vi "Test Executable.vi"() -> ()   [LabVIEW 2014]
uses:
  Core/LabVIEW CI Service/Classes/LabVIEW Instance/LabVIEW Instance.lvclass
  Dummy Job/Dummy Job.lvclass
  Core/LabVIEW CI Service/Actors/Jobber Proxy/Jobber Proxy/Jobber Proxy.lvclass
  <vilib>/ActorFramework/Actor/Actor.lvclass
  <vilib>/ActorFramework/Message Queue/Message Queue.lvclass
  <vilib>/ActorFramework/Message Dequeuer/Message Dequeuer.lvclass
  <vilib>/ActorFramework/LastAck/Last Ack.lvclass
  Core/LabVIEW CI Service/Classes/Job/Job.lvclass
  Core/LabVIEW CI Service/Controls/Job Results - STYP.ctl
panel:
  out "Boolean":bool
  in  "Wait (ms)":u32=30000
  out "Results":T1 {"Status" items=["Service Error"=504, "Abort"=503, "Fail"=500, "Pass"=200]}
  in  "Launch":bool
  in  "Show Panel":bool=TRUE
  in  "Open":bool
  in  "Port":i32=3366
  in  "Machine Name":string="10.0.19.177"
  in  "stop":bool
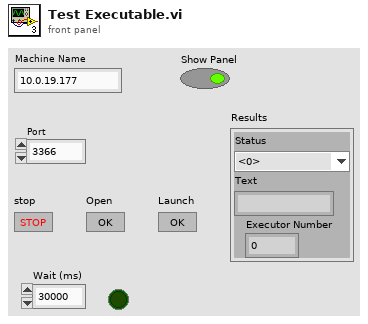
[diagram p1: front panel]
types:
  T1 = typedef "Job Results - STYP.ctl" = cluster{"Status":u16, "Text":string, "Executor Number":i32}
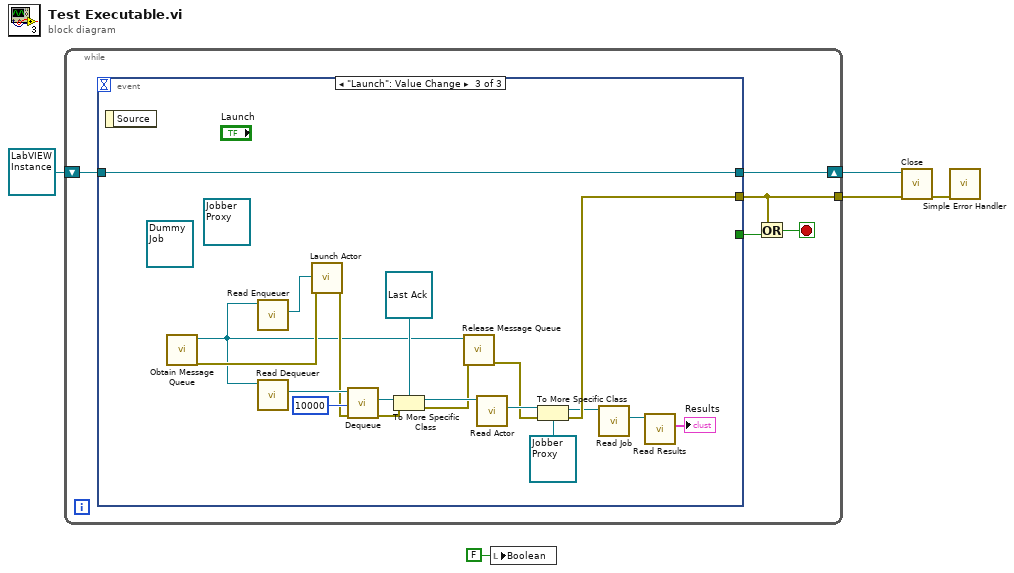
[diagram p0: block diagram]
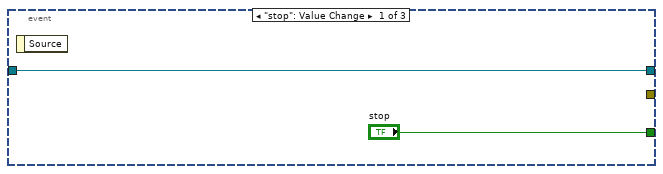
[diagram p2: hidden frame]
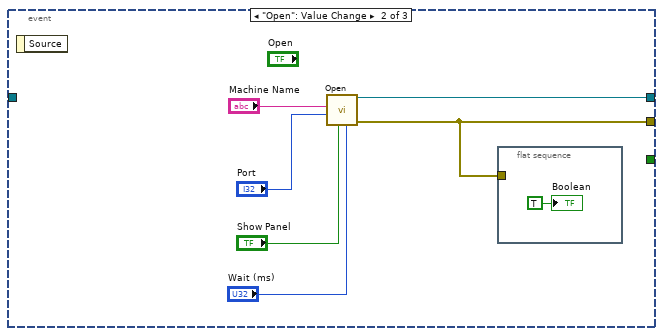
[diagram p3: hidden frame]
diagram:
  n1 = while {
    shift-right: [w9] -> w4
    shift-left: refnum<class "LabVIEW Instance.lvclass"> refnum ("LabVIEW Instance") -> [w10]
    tunnel: [w8] -> w2
    stop <- w7 stop-if-true
    n2 = event shown="[2] \"Launch\": Value Change" {
      selector: _ -> [_ _ _]
      dyn-events: _ -> [_ _ _]
      timeout: _ -> [_ _ _]
      tunnel: w10 -> [w12 _ w38]
      tunnel: [w12 w16 w38] -> w9
      tunnel: [_ w13 w24] -> w8
      tunnel: ["stop" _ _] -> w6
      event "stop": Value Change {
        n3 = event-data() -> ()  [unwired: 1 in, 1 out]
      }
      event "Open": Value Change {
        n4 = event-data() -> ()  [unwired: 1 in, 1 out]
        n5 = call "Open.vi"("Wait"="Wait (ms)", "Show Panel"="Show Panel", 9:"Port", 10:"Machine Name") -> ("error out"=w13:errorcluster, "LabVIEW Instance"=w16:refnum<class "LabVIEW Instance.lvclass">)  [unwired: 6 in]
        n6 = flat-sequence {
          tunnel: w13 -> [_]
          frame #0 {
            "Boolean" <- TRUE ("Boolean")
          }
        }
      }
      event "Launch": Value Change {
        (unwired) refnum<class "Jobber Proxy.lvclass"> refnum ("Jobber Proxy in")
        (unwired) refnum<class "Dummy Job.lvclass"> refnum ("Dummy Job.lvclass")
        n7 = event-data() -> ()  [unwired: 1 in, 1 out]
        n8 = call <vilib>:"Obtain Message Queue.vi"() -> ("error out"=w36:errorcluster, "Message Queue"=w27:refnum<class "Message Queue.lvclass">)  [unwired: 10 in]
        n9 = call <vilib>:"Read Enqueuer.vi"("Message Queue"=w27) -> ("Message Enqueuer"=w37:refnum<class "Message Enqueuer.lvclass">)  [unwired: 10 in]
        n10 = call <vilib>:"Read Dequeuer.vi"("Message Queue"=w27) -> ("Message Dequeuer"=w35:refnum<class "Message Dequeuer.lvclass">)  [unwired: 10 in]
        n11 = call <vilib>:"Launch Actor.vi"("error in (no error)"=w36, "Actor-to-Caller Enqueuer"=w37) -> ("error out"=w33:errorcluster)  [unwired: 8 in, 1 out]
        n12 = call <vilib>:"Dequeue.vi"("error in (no error)"=w33, "timeout in ms (-1)"=10000, "Message Dequeuer in"=w35) -> ("error out"=w31:errorcluster, "Message"=w32:refnum<class "Message.lvclass">)  [unwired: 4 in, 3 out]
        n13 = To More Specific Class(target class=refnum<class "Last Ack.lvclass"> refnum ("Last Ack"), reference=w32, error in=w31) -> (specific class reference=w30:refnum<class "Last Ack.lvclass">, error out=w28:errorcluster)
        n14 = call <vilib>:"Release Message Queue.vi"("error in (no error)"=w28, "Message Queue"=w27) -> ("error out"=w23:errorcluster)  [unwired: 8 in, 1 out]
        n15 = call <vilib>:"Read Actor.vi"("Last Ack"=w30) -> ("Actor"=w26:refnum<class "Actor.lvclass">)  [unwired: 10 in]
        n16 = To More Specific Class(target class=refnum<class "Jobber Proxy.lvclass"> refnum ("Jobber Proxy.lvlib:Jobber Proxy.lvclass"), reference=w26, error in=w23) -> (specific class reference=w21:refnum<class "Jobber Proxy.lvclass">, error out=w24:errorcluster)
        n17 = call "Read Job.vi"("Jobber Proxy in"=w21) -> ("Job"=w20:refnum<class "Job.lvclass">)  [unwired: 10 in]
        n18 = call "Read Results.vi"("Job in"=w20) -> ("Results"=→"Results":T1)  [unwired: 10 in]
      }
    }
    n19 = Or(x=w8, y=w6) -> (x .or. y?=w7:bool)
  }
  n20 = local write "Boolean"(FALSE ("Boolean")) -> ()
  n21 = call "Close.vi"("error in (no error)"=w2, "LabVEIW Instance in"=w4) -> ("error out"=w3:errorcluster)  [unwired: 9 in]
  n22 = call <vilib>:"Simple Error Handler.vi"("error in (no error)"=w3) -> ()  [unwired: 4 in, 5 out]
